vi "Insert Element in Trace for Tag.vi"(6 "error in (no error)":errorcluster, 10 "Tag in":refnum<class "Tag.lvclass">, 11 "TraceLength":i32=10) -> (4 "error out":errorcluster)   [LabVIEW 2014, in "Tag.lvclass"]
doc: "This VI pushes a new element (XY coordinate) to the array of traces for a Tag.\nAs a result the output is a collection of traces of length = TraceLength."
uses:
  Tag.lvclass
panel:
  out "Trace Out":cluster{dbl[], dbl[]}[][](array[cluster])
  in  "Array":cluster{"x":dbl[], "y":dbl[]}[](array[cluster])
  in  "ElementX":dbl format="%#_13g"
  in  "ElementY":dbl format="%#_13g"
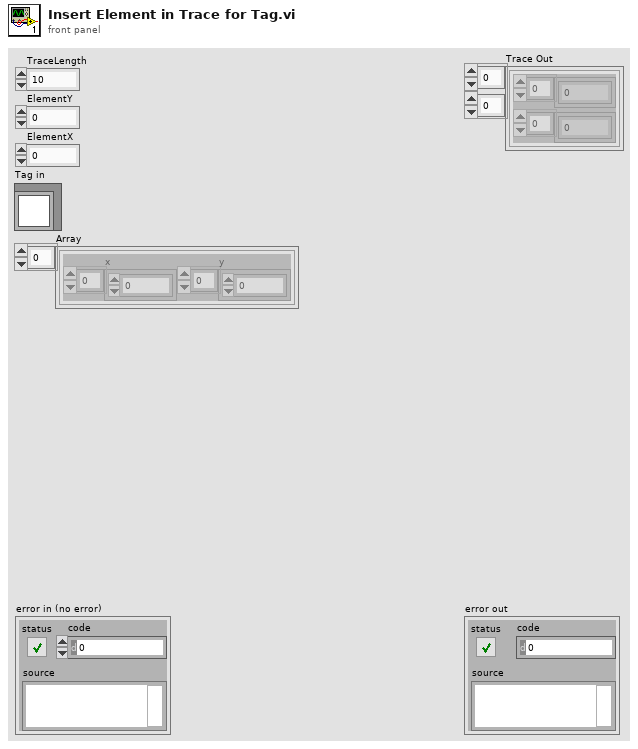
[diagram p1: front panel]
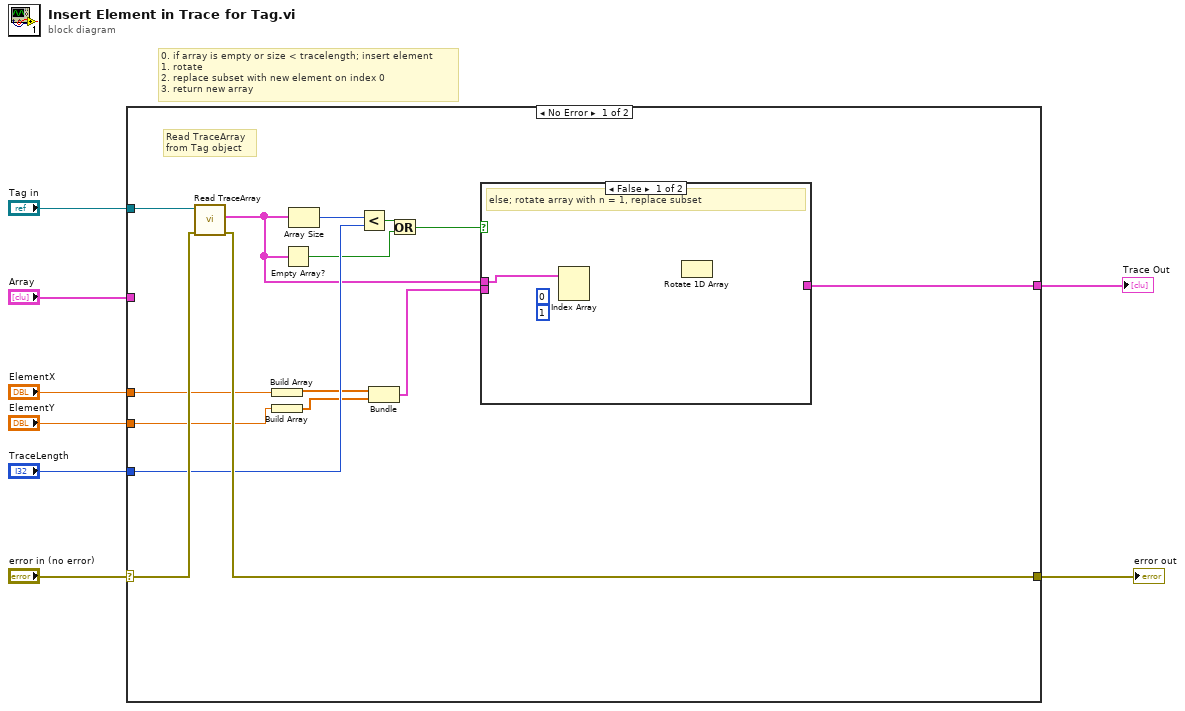
[diagram p0: block diagram]
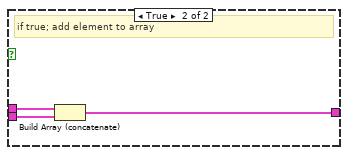
[diagram p2: hidden frame]
diagram:
  # "0. if array is empty or size < tracelength; insert element\n1. rotate\n2. replace subset with new element on index 0\n3. return new array"
  n1 = case shown="No Error" "error in (no error)" {
    selector: "error in (no error)" -> [w22 w28]
    tunnel: [w21 w28] -> w7
    tunnel: "Tag in" -> [w23 _]
    tunnel: "Array" -> [_ _]
    tunnel: "ElementY" -> [w13 _]
    tunnel: "ElementX" -> [w14 _]
    tunnel: "TraceLength" -> [w19 _]
    tunnel: [w9 _] -> w1
    frame No Error {
      # "Read TraceArray\nfrom Tag object"
      n2 = call-dynamic "Read TraceArray.vi"("error in (no error)"=w22, "Tag in"=w23) -> ("error out"=w21:errorcluster, "TraceArray"=w15:cluster{dbl[], dbl[]}[])  [unwired: 7 in, 1 out]
      n3 = Build Array(w14) -> (w12:dbl[])
      n4 = Build Array(w13) -> (w11:dbl[])
      n5 = Empty Array?(array=w15) -> (empty?=w17:bool)
      n6 = Array Size(array=w15) -> (size(s)=w20:i32)
      n7 = Less?(x=w20, y=w19) -> (x < y?=w18:bool)
      n8 = Bundle(w12, w11) -> (w10:cluster{dbl[], dbl[]})  [unwired: 1 in]
      n9 = Or(x=w18, y=w17) -> (x .or. y?=w16:bool)
      n10 = case shown="False" w16 {
        tunnel: w15 -> [w24 w27]
        tunnel: w10 -> [_ w26]
        tunnel: [_ w25] -> w9
        frame False {
          (unwired) 1 ("index (col)")
          (unwired) 0 ("disabled index (col)")
          # "else; rotate array with n = 1, replace subset"
          n11 = Index Array(array=w24) -> ()  [unwired: 2 in, 2 out]
          n12 = Rotate 1D Array() -> ()  [unwired: 2 in, 1 out]
        }
        frame True {
          # "if true; add element to array"
          n13 = Build Array (concatenate)(w27, w26) -> (w25:cluster{dbl[], dbl[]}[])
        }
      }
    }
    frame Error {
    }
  }
  "error out" <- w7
  "Trace Out" <- w1
